vi "Get Setpoint.vi"(10 "Point":string, 11 "Task Base in":refnum<class "Task Base.lvclass">) -> (1 "Value":variant, 2 "found?":bool, 3 "Task Base out":refnum<class "Task Base.lvclass">)   [LabVIEW 2023, in "Task Base.lvclass"]
uses:
  Task Base.lvclass
  Task Base.lvclass/Task Base.ctl
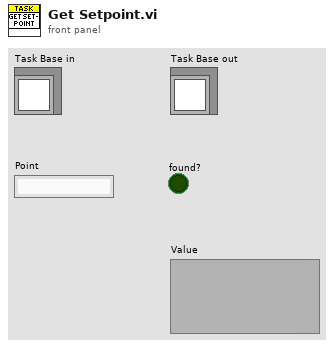
[diagram p1: front panel]
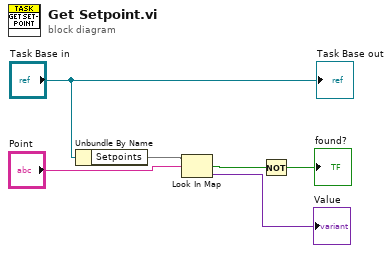
[diagram p0: block diagram]
diagram:
  n1 = Unbundle By Name("Task Base in") -> ("Setpoints"=w5:map{string, variant})
  n2 = Look In Map(map=w5, key="Point") -> (key not found?=w3:bool, value=→"Value":variant)  [unwired: 1 in]
  n3 = Not(x=w3) -> (.not. x?=→"found?":bool)
  "Task Base out" <- "Task Base in"
